vi "Get INFO from ini FILE - SRTRS.vi"(0 "ini Name":string="MyEXE.ini", 5 "Application Directory (Default if blank)":path, 11 "Error In":errorcluster) -> (1 "Settings":T5, 2 "Equipment Details (MCListBox)":string[][](array[string]), 3 "Furnace Details":T4, 4 "ini Path":path=path "C:/Users/CK/workspace/LabVIEW/Configuration File Test/MyEXE.ini", 6 "SRTRS Connection Information":T1={"Connection "="SQL Server 32bit HPEnvy", "Username"="admin", "Password"="admin123"}, 8 "CMS Connection Information":T1={"Connection "="SQL Server 32bit HPEnvy", "Username"="admin", "Password"="admin123"}, 10 "AMS Connection Information":T1={"Connection "="SQL Server 32bit HPEnvy", "Username"="admin", "Password"="admin123"}, 12 "MessageQ":string, 14 "Settings Boolean":T2, 15 "Error Out":errorcluster)   [LabVIEW 2013]
uses:
  Controls/Connection Information Cluster.ctl
  <vilib>/Utility/config.llb/Read Key (String).vi
  <vilib>/Utility/config.llb/Read Key (Boolean).vi
  <vilib>/Utility/config.llb/NI_LVConfig.lvlib
  <vilib>/Utility/config.llb/Write Key (I32).vi
panel:
  out "Equipment Details":T3
  out "Application Directory":path=path "C:/Users/CK/workspace/LabVIEW/Configuration File Test"
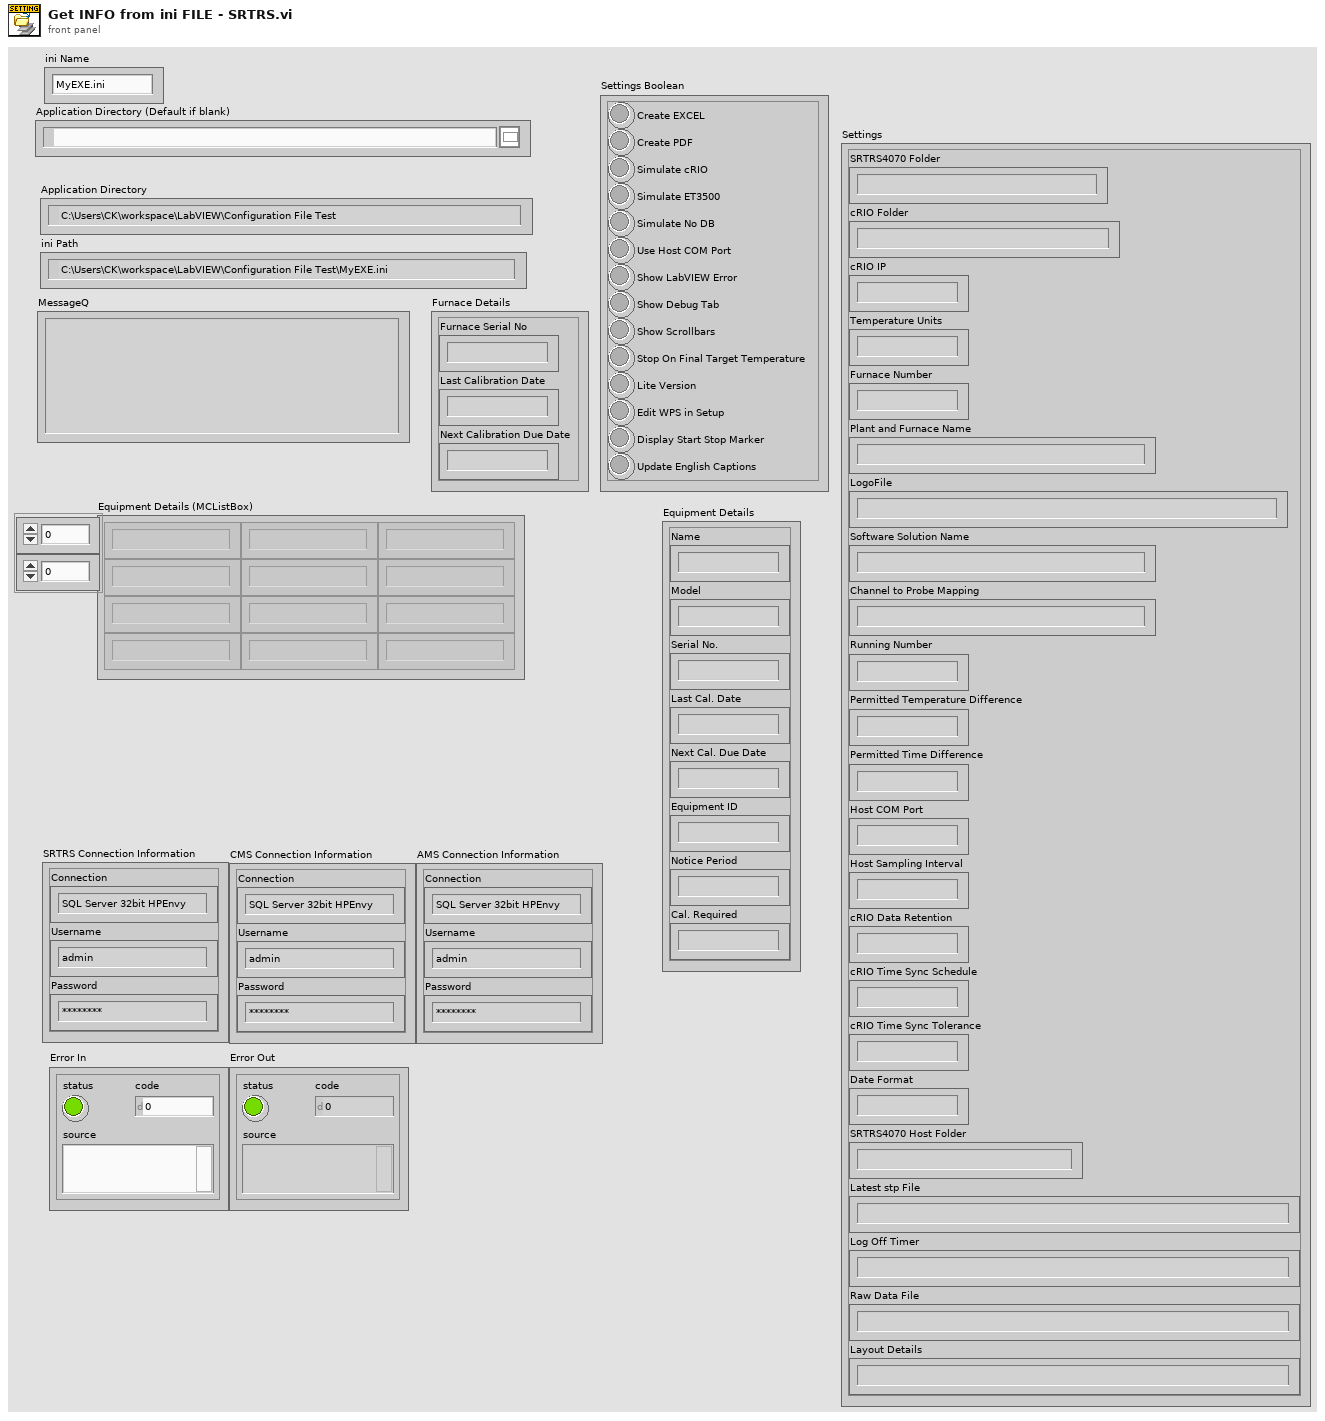
[diagram p1: front panel]
types:
  T1 = typedef "Connection Information Cluster.ctl" = cluster{"Connection ":string, "Username":string, "Password":string}
  T2 = cluster{"Create EXCEL":bool, "Create PDF":bool, "Simulate cRIO":bool, "Simulate ET3500":bool, "Simulate No DB":bool, "Use Host COM Port":bool, "Show LabVIEW Error":bool, "Show Debug Tab":bool, "Show Scrollbars":bool, "Stop On Final Target Temperature":bool, "Lite Version":bool, "Edit WPS in Setup":bool, "Display Start Stop Marker":bool, "Update English Captions":bool}
  T3 = cluster{"Name":string, "Model":string, "Serial No.":string, "Last Cal. Date":string, "Next Cal. Due Date":string, "Equipment ID":string, "Notice Period":string, "Cal. Required":string}
  T4 = cluster{"Furnace Serial No":string, "Last Calibration Date":string, "Next Calibration Due Date":string}
  T5 = cluster{"SRTRS4070 Folder":string, "cRIO Folder":string, "cRIO IP":string, "Temperature Units":string, "Furnace Number":string, "Plant and Furnace Name":string, "LogoFile":string, "Software Solution Name":string, "Channel to Probe Mapping":string, "Running Number":string, "Permitted Temperature Difference":string, "Permitted Time Difference":string, "Host COM Port":string, "Host Sampling Interval":string, "cRIO Data Retention":string, "cRIO Time Sync Schedule":string, "cRIO Time Sync Tolerance":string, "Date Format":string, "SRTRS4070 Host Folder":string, "Latest stp File":string, "Log Off Timer":string, "Raw Data File":string, "Layout Details":string}
  T6 = typedef "NI_LVConfig.lvlib/Config Data RefNum.ctl" = refnum<k1>
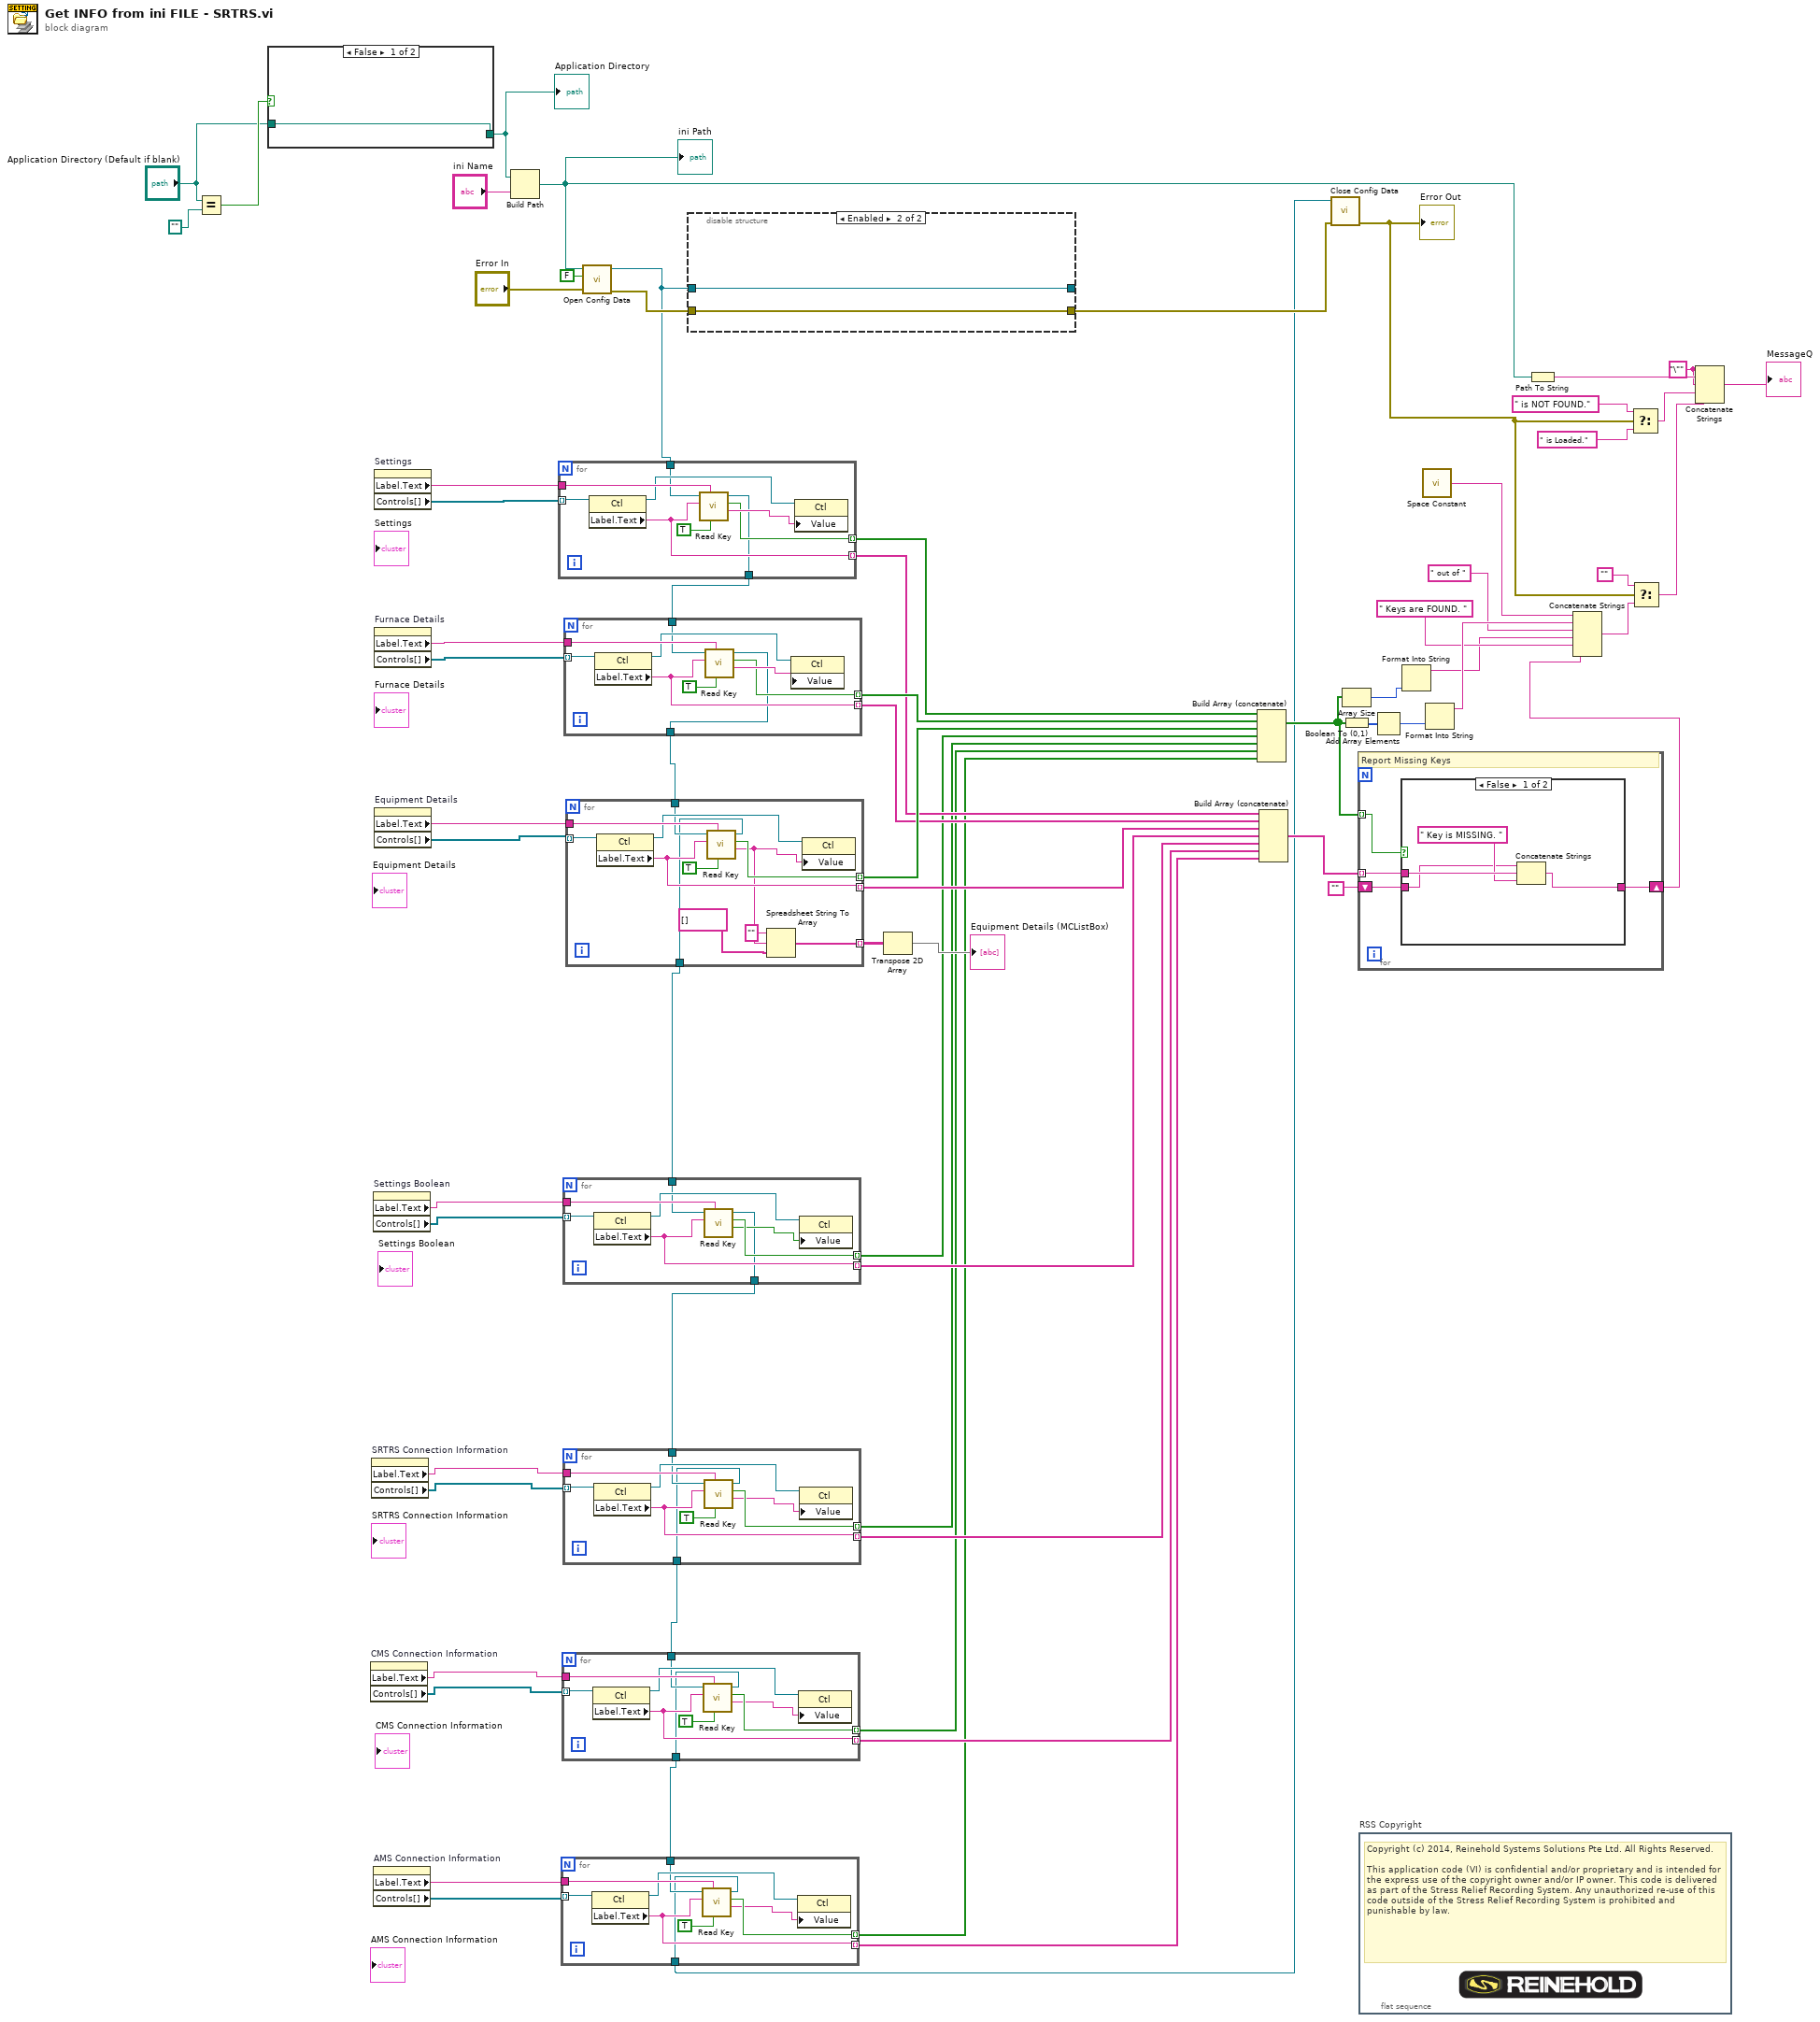
[diagram p0: block diagram]
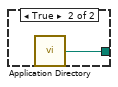
[diagram p2: hidden frame]
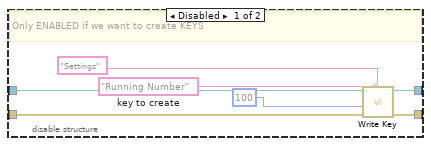
[diagram p4: hidden frame]
diagram:
  w64 = "\"" ("string")
  n1 = Equal?(x="Application Directory (Default if blank)", y=path "") -> (x = y?=w42:bool)
  n2 = case shown="False" w42 {
    tunnel: [w71 w72] -> w70
    tunnel: "Application Directory (Default if blank)" -> [w71 _]
    frame False {
    }
    frame True {
      n3 = call <vilib>:"Application Directory.vi"() -> ("Application Directory"=w72:path)
    }
  }
  "Application Directory" <- w70
  n4 = property on="CMS Connection Information" class="Clust (strict)"() -> ("Label.Text"=w12:string, "Controls[]"=w13:refnum<vi>[])  [unwired: 2 in, 2 out]
  n5 = property on="SRTRS Connection Information" class="Clust (strict)"() -> ("Label.Text"=w17:string, "Controls[]"=w16:refnum<vi>[])  [unwired: 2 in, 2 out]
  n6 = property on="Settings Boolean" class="Clust (strict)"() -> ("Label.Text"=w18:string, "Controls[]"=w22:refnum<vi>[])  [unwired: 2 in, 2 out]
  n7 = property on="AMS Connection Information" class="Clust (strict)"() -> ("Label.Text"=w9:string, "Controls[]"=w8:refnum<vi>[])  [unwired: 2 in, 2 out]
  n8 = property on="Settings" class="Clust (strict)"() -> ("Label.Text"=w38:string, "Controls[]"=w39:refnum<vi>[])  [unwired: 2 in, 2 out]
  n9 = property on="Furnace Details" class="Clust (strict)"() -> ("Label.Text"=w37:string, "Controls[]"=w36:refnum<vi>[])  [unwired: 2 in, 2 out]
  n10 = property on="Equipment Details" class="Clust (strict)"() -> ("Label.Text"=w23:string, "Controls[]"=w35:refnum<vi>[])  [unwired: 2 in, 2 out]
  n11 = Build Path(base path=w70, name or relative path="ini Name") -> (appended path=w66:path)
  "ini Path" <- w66
  n12 = call <vilib>:"Open Config Data.vi"("error in (no error)"="Error In", "create file if necessary (T)"=FALSE, "configuration file path"=w66) -> ("error out"=w67:errorcluster, "refnum"=w26:T6)  [unwired: 6 in, 1 out]
  n13 = for {
    tunnel: w39 -> [w81] mode=indexing
    tunnel: w38 -> [w80]
    tunnel: [w77] -> w34 mode=indexing
    tunnel: w26 -> [w76]
    tunnel: [w75] -> w31 mode=indexing
    tunnel: [w74] -> w28
    n14 = property class="Ctl"(reference=w81) -> (reference out=w79:refnum<vi>, "Label.Text"=w75:string)  [unwired: 1 in, 1 out]
    n15 = call-poly <vilib>:"Read Key.vi"("read raw string? (F)"=TRUE, "section"=w80, "key"=w75, "refnum"=w76) -> ("value"=w78:string, "found?"=w77:bool, "refnum out"=w74:T6)  [unwired: 4 in, 1 out]
    n16 = property class="Ctl"(reference=w79, "Value"=w78) -> ()  [unwired: 1 in, 2 out]
  }
  n17 = for {
    tunnel: w36 -> [w90] mode=indexing
    tunnel: w37 -> [w89]
    tunnel: [w86] -> w33 mode=indexing
    tunnel: w28 -> [w85]
    tunnel: [w84] -> w30 mode=indexing
    tunnel: [w83] -> w27
    n18 = property class="Ctl"(reference=w90) -> (reference out=w88:refnum<vi>, "Label.Text"=w84:string)  [unwired: 1 in, 1 out]
    n19 = call-poly <vilib>:"Read Key.vi"("read raw string? (F)"=TRUE, "section"=w89, "key"=w84, "refnum"=w85) -> ("value"=w87:string, "found?"=w86:bool, "refnum out"=w83:T6)  [unwired: 4 in, 1 out]
    n20 = property class="Ctl"(reference=w88, "Value"=w87) -> ()  [unwired: 1 in, 2 out]
  }
  n21 = for {
    tunnel: w35 -> [w102] mode=indexing
    tunnel: w23 -> [w101]
    tunnel: [w99] -> w32 mode=indexing
    tunnel: w27 -> [w98]
    tunnel: [w97] -> w29 mode=indexing
    tunnel: [w93] -> w25 mode=indexing
    tunnel: [w92] -> w1
    n22 = property class="Ctl"(reference=w102) -> (reference out=w100:refnum<vi>, "Label.Text"=w97:string)  [unwired: 1 in, 1 out]
    n23 = call-poly <vilib>:"Read Key.vi"("read raw string? (F)"=TRUE, "section"=w101, "key"=w97, "refnum"=w98) -> ("value"=w96:string, "found?"=w99:bool, "refnum out"=w92:T6)  [unwired: 4 in, 1 out]
    n24 = Spreadsheet String To Array(format string="", spreadsheet string=w96, array type (2D Dbl)=string[] []) -> (array=w93:string[])  [unwired: 1 in]
    n25 = property class="Ctl"(reference=w100, "Value"=w96) -> ()  [unwired: 1 in, 2 out]
  }
  n26 = for {
    tunnel: w22 -> [w110] mode=indexing
    tunnel: w18 -> [w109]
    tunnel: [w107] -> w20 mode=indexing
    tunnel: w1 -> [w106]
    tunnel: [w105] -> w21 mode=indexing
    tunnel: [w103] -> w2
    n27 = property class="Ctl"(reference=w110) -> (reference out=w108:refnum<vi>, "Label.Text"=w105:string)  [unwired: 1 in, 1 out]
    n28 = call-poly <vilib>:"Read Key.vi"("section"=w109, "key"=w105, "refnum"=w106) -> ("value"=w104:bool, "found?"=w107:bool, "refnum out"=w103:T6)  [unwired: 5 in, 1 out]
    n29 = property class="Ctl"(reference=w108, "Value"=w104) -> ()  [unwired: 1 in, 2 out]
  }
  n30 = for {
    tunnel: w16 -> [w119] mode=indexing
    tunnel: w17 -> [w118]
    tunnel: [w116] -> w15 mode=indexing
    tunnel: w2 -> [w115]
    tunnel: [w114] -> w14 mode=indexing
    tunnel: [w112] -> w11
    n31 = property class="Ctl"(reference=w119) -> (reference out=w117:refnum<vi>, "Label.Text"=w114:string)  [unwired: 1 in, 1 out]
    n32 = call-poly <vilib>:"Read Key.vi"("read raw string? (F)"=TRUE, "section"=w118, "key"=w114, "refnum"=w115) -> ("value"=w113:string, "found?"=w116:bool, "refnum out"=w112:T6)  [unwired: 4 in, 1 out]
    n33 = property class="Ctl"(reference=w117, "Value"=w113) -> ()  [unwired: 1 in, 2 out]
  }
  n34 = for {
    tunnel: w13 -> [w128] mode=indexing
    tunnel: w12 -> [w127]
    tunnel: [w125] -> w5 mode=indexing
    tunnel: w11 -> [w124]
    tunnel: [w123] -> w10 mode=indexing
    tunnel: [w121] -> w7
    n35 = property class="Ctl"(reference=w128) -> (reference out=w126:refnum<vi>, "Label.Text"=w123:string)  [unwired: 1 in, 1 out]
    n36 = call-poly <vilib>:"Read Key.vi"("read raw string? (F)"=TRUE, "section"=w127, "key"=w123, "refnum"=w124) -> ("value"=w122:string, "found?"=w125:bool, "refnum out"=w121:T6)  [unwired: 4 in, 1 out]
    n37 = property class="Ctl"(reference=w126, "Value"=w122) -> ()  [unwired: 1 in, 2 out]
  }
  n38 = for {
    tunnel: w8 -> [w137] mode=indexing
    tunnel: w9 -> [w136]
    tunnel: [w134] -> w4 mode=indexing
    tunnel: w7 -> [w133]
    tunnel: [w132] -> w3 mode=indexing
    tunnel: [w130] -> w6
    n39 = property class="Ctl"(reference=w137) -> (reference out=w135:refnum<vi>, "Label.Text"=w132:string)  [unwired: 1 in, 1 out]
    n40 = call-poly <vilib>:"Read Key.vi"("read raw string? (F)"=TRUE, "section"=w136, "key"=w132, "refnum"=w133) -> ("value"=w131:string, "found?"=w134:bool, "refnum out"=w130:T6)  [unwired: 4 in, 1 out]
    n41 = property class="Ctl"(reference=w135, "Value"=w131) -> ()  [unwired: 1 in, 2 out]
  }
  n42 = disable-structure shown="Enabled" {
    disable-tunnel: w67 -> [w144 w145]
    disable-tunnel: [w141 w145] -> w19
    disable-tunnel: [w142 w146] -> _
    disable-tunnel: w26 -> [w143 w146]
    frame Disabled {
      w140 = "Running Number"  # key to create
      # "Only ENABLED if we want to create KEYS"
      n43 = call-poly <vilib>:"Write Key.vi"("section"="Settings", "error in (no error)"=w144, "value"=100 ("default value"), "key"=w140, "refnum"=w143) -> ("error out"=w141:errorcluster, "refnum out"=w142:T6)  [unwired: 4 in, 1 out]
    }
    frame Enabled {
    }
  }
  n44 = Transpose 2D Array(2D array=w25) -> (transposed array=→"Equipment Details (MCListBox)":string[][])
  n45 = Build Array (concatenate)(w34, w33, w32, w20, w15, w5, w4) -> (w46:bool[])
  n46 = Build Array (concatenate)(w31, w30, w29, w21, w14, w10, w3) -> (w40:string[])
  n47 = call <vilib>:"Close Config Data.vi"("error in (no error)"=w19, "refnum"=w6) -> ("error out"=w50:errorcluster)  [unwired: 8 in, 1 out]
  "Error Out" <- w50
  n48 = Array Size(array=w46) -> (size(s)=w45:i32)
  n49 = Boolean To (0,1)(Boolean=w46) -> (0, 1=w59:i16[])
  n50 = for {
    tunnel: w46 -> [w150] mode=indexing
    tunnel: w40 -> [w149] mode=indexing
    shift-right: [w147] -> w48
    shift-left: "" -> [w148]
    # "Report Missing Keys"
    n51 = case shown="False" w150 {
      tunnel: w149 -> [w154 _]
      tunnel: w148 -> [w152 w155]
      tunnel: [w151 w155] -> w147
      frame False {
        n52 = Concatenate Strings(w152, w154, " Key is MISSING. " ("string")) -> (w151:string)
      }
      frame True {
      }
    }
  }
  n53 = flat-sequence "RSS Copyright" {
    frame #0 {
      # "Copyright (c) 2014, Reinehold Systems Solutions Pte Ltd. All Rights Reserved.\n\nThis application code (VI) is confidential and/or proprietary and is intended for the express use of the copyright owner and/or IP owner. This code is delivered as part of the Stress Relief Recording System. Any unauthorized re-use of this code outside of the Stress Relief Recording System is prohibited and punishable by law."
    }
  }
  n54 = Add Array Elements(numeric array=w59) -> (sum=w58:i16)
  n55 = Format Into String(w45) -> (resulting string=w44:string)  [unwired: 3 in, 1 out]
  n56 = call <vilib>:"Space Constant.vi"() -> ("String"=w56:string)
  n57 = Format Into String(w58) -> (resulting string=w55:string)  [unwired: 3 in, 1 out]
  n58 = Path To String(path=w66) -> (string=w65:string)
  n59 = Concatenate Strings(w56, w55, " out of " ("string"), w44, " Keys are FOUND. " ("string"), w48) -> (w53:string)
  n60 = Select(t=" is NOT FOUND." ("string"), s=w50, f=" is Loaded." ("string")) -> (s? t:f=w62:string)
  n61 = Select(t="", s=w50, f=w53) -> (s? t:f=w52:string)
  n62 = Concatenate Strings(w64, w65, w64, w62, w52) -> (→"MessageQ":string)
